vi "Run Test.vi"(8 "error in (no error)":errorcluster, 11 "Test Template in":refnum<class "Temp Soak.lvclass">) -> (0 "error out":errorcluster, 1 "Positions":i32[](array[numeric]), 2 "Tests Passed":bool[](array[boolean]), 3 "Test Template out":refnum<class "Temp Soak.lvclass">, 5 "Fail Codes":string[](array[string]))   [LabVIEW 2015, in "Temp Soak.lvclass"]
uses:
  Temp Soak.lvclass
  CBTF Applications/Reliability Testing/Main/Rel Load Curve Tracer/Application/Application/Class/typedefs/Instrument Selector -- Enum.ctl
  Classes/Instruments/Temperature Device/ThorLabs TSP01/Class/ThorLabs TSP01.lvclass
  Classes/Instruments/DC Power Supply/DC Power Supply/Class/DC Power Supply.lvclass
  Test Class/Test Class.lvclass
  Classes/Application/Class/Application.lvclass
  CBTF Applications/Reliability Testing/Main/Rel Load Curve Tracer/Application/Application/Class/Rel Curve Tracer.lvclass
panel:
  out "Target Temperature":dbl format="%.3f"
  out "Actual Temperature":dbl format="%.3f"
  # "Please wait for Temperature Soak completion."
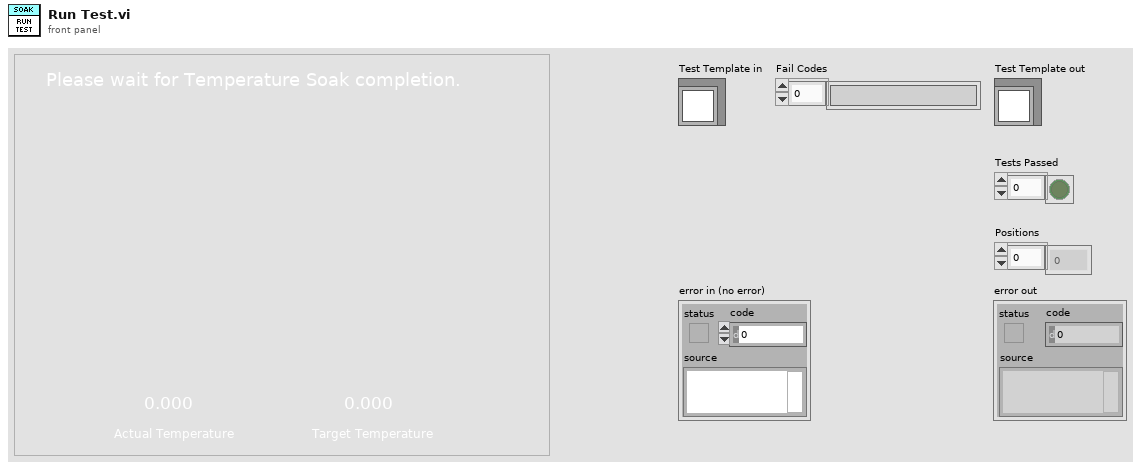
[diagram p1: front panel]
types:
  T1 = typedef "Rel Curve Tracer.lvlib/Rel Curve Tracer.lvclass/Instrument Selector -- Enum.ctl" = enum16{"DC Power Supply", "Temp Device", "Switch"}
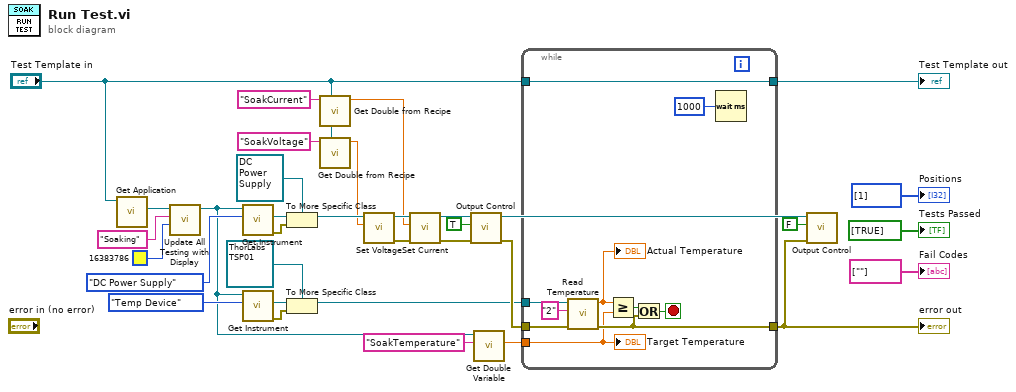
[diagram p0: block diagram]
diagram:
  n1 = call "Get Application.vi"("Test Class in"="Test Template in") -> ("Application.lvlib:Application.lvclass"=w33:refnum<class "Application.lvclass">)  [unwired: 9 in, 1 out]
  n2 = call "Update All Testing with Display.vi"("BG Color"=u32 16383786, "Message ('')"="Soaking", "Application in"=w33) -> ("Application out"=w4:refnum<class "Application.lvclass">)  [unwired: 7 in, 1 out]
  n3 = call "Get Instrument.vi"("Instrument Number"=Instrument_Selector_--_Enum."DC Power Supply" ("Instrument"), "Application in"=w4) -> ("error out"=w26:errorcluster, "Instrument"=w29:refnum<class "Instrument.lvclass">)  [unwired: 7 in, 1 out]
  n4 = call "Get Instrument.vi"("Instrument Number"=Instrument_Selector_--_Enum."Temp Device" ("Instrument"), "Application in"=w4) -> ("error out"=w27:errorcluster, "Instrument"=w28:refnum<class "Instrument.lvclass">)  [unwired: 7 in, 1 out]
  n5 = To More Specific Class(target class=refnum<class "DC Power Supply.lvclass"> refnum ("DC Power Supply.lvlib:DC Power Supply.lvclass"), reference=w29, error in=w26) -> (specific class reference=w24:refnum<class "DC Power Supply.lvclass">)  [unwired: 1 out]
  n6 = To More Specific Class(target class=refnum<class "ThorLabs TSP01.lvclass"> refnum ("ThorLabs TSP01.lvlib:ThorLabs TSP01.lvclass"), reference=w28, error in=w27) -> (specific class reference=w12:refnum<class "ThorLabs TSP01.lvclass">)  [unwired: 1 out]
  n7 = call "Get Double from Recipe.vi"("Test Class in"="Test Template in", "Name"="SoakCurrent") -> ("Value"=w7:dbl)  [unwired: 7 in, 2 out]
  n8 = call "Get Double from Recipe.vi"("Test Class in"="Test Template in", "Name"="SoakVoltage") -> ("Value"=w6:dbl)  [unwired: 7 in, 2 out]
  n9 = call-dynamic "Set Voltage.vi"("Voltage (0.0 V)"=w6, "Acrobat Template in"=w24) -> ("error out"=w22:errorcluster, "Acrobat Template out"=w23:refnum<class "DC Power Supply.lvclass">)  [unwired: 8 in]
  n10 = call-dynamic "Set Current.vi"("error in (no error)"=w22, "Current (0.0A)"=w7, "Acrobat Template in"=w23) -> ("error out"=w16:errorcluster, "Acrobat Template out"=w17:refnum<class "DC Power Supply.lvclass">)  [unwired: 7 in]
  n11 = call-dynamic "Output Control.vi"("error in (no error)"=w16, "Enabled"=TRUE, "Acrobat Template in"=w17) -> ("error out"=w15:errorcluster, "Acrobat Template out"=w10:refnum<class "DC Power Supply.lvclass">)  [unwired: 7 in]
  n12 = call "Get Double Variable.vi"("Name"="SoakTemperature", "Application in"=w4) -> ("Value"=w3:dbl)  [unwired: 7 in, 2 out]
  n13 = while {
    tunnel: w15 -> [w40]
    tunnel: [w37] -> w11
    tunnel: [w41] -> w19
    tunnel: "Test Template in" -> [w41]
    tunnel: w12 -> [w44]
    tunnel: w3 -> [w35]
    stop <- w36 stop-if-true
    n14 = call-dynamic "Read Temperature.vi"("error in (no error)"=w40, "Channel"="2", "Acrobat Template in"=w44) -> ("error out"=w37:errorcluster, "Temperature out"=w39:dbl)  [unwired: 7 in]
    "Actual Temperature" <- w39
    n15 = Greater Or Equal?(x=w39, y=w35) -> (x >= y?=w38:bool)
    n16 = Or(x=w38, y=w37) -> (x .or. y?=w36:bool)
    n17 = Wait (ms)(milliseconds to wait=u32 1000) -> ()  [unwired: 1 out]
    "Target Temperature" <- w35
  }
  "error out" <- w11
  "Test Template out" <- w19
  n18 = call-dynamic "Output Control.vi"("error in (no error)"=w11, "Enabled"=FALSE, "Acrobat Template in"=w10) -> ()  [unwired: 7 in, 2 out]
  "Tests Passed" <- bool[] [TRUE] ("Tests Passed")
  "Fail Codes" <- string[] [""] ("Fail Codes")
  "Positions" <- i32[] [1] ("Positions")
